vi "Демультиплексор-5-разр.vi"(1 "c 1":bool, 2 "c 0":bool, 3 "?":bool) -> (0 "Out":T1)   [LabVIEW 2012]
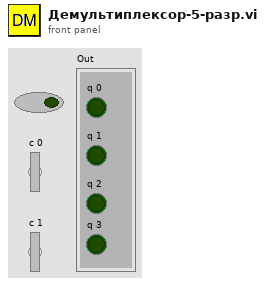
[diagram p1: front panel]
types:
  T1 = cluster{"q 0":bool, "q 1":bool, "q 2":bool, "q 3":bool}
  T2 = cluster{" 1":bool, "2":bool, " 1":bool, "2":bool}
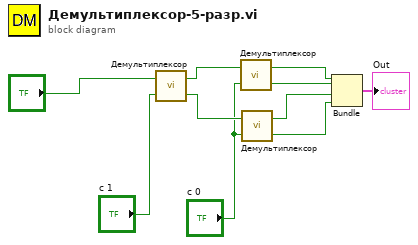
[diagram p0: block diagram]
diagram:
  n1 = call "Демультиплексор.vi"(2:"c 1", 3:"?") -> ("2"=w7:bool, "1"=w8:bool)
  n2 = call "Демультиплексор.vi"(2:"c 0", 3:w8) -> ("2"=w5:bool, "1"=w6:bool)
  n3 = call "Демультиплексор.vi"(2:"c 0", 3:w7) -> ("2"=w3:bool, "1"=w4:bool)
  n4 = Bundle("1"=w6, "2"=w5, "1"=w4, "2"=w3) -> (→"Out":T2)  [unwired: 1 in]
